vi "ChoixFiltres.vi"(1 "Ordre des filtres Avant":string[](array[string])=["Aucun filtre", "Filtre 1", "Filtre 2", "Filtre 3", "Filtre 4", ""]) -> (0 "Ordre des filtres Après":string[](array[string])=["Aucun filtre", "Filtre 1", "Filtre 2", "Filtre 3", "Filtre 4", ""])   [LabVIEW 2011]
panel:
  in  "Annuler":bool
  in  "OK":bool
  in  "Filtre 6":string
  in  "Filtre 5":string="Filtre 4"
  in  "Filtre 4":string="Filtre 3"
  in  "Filtre 3":string="Filtre 2"
  in  "Filtre 2":string="Filtre 1"
  in  "Filtre 1":string="Aucun filtre"
  # "Appuyer sur \"ENTER\" pour confirmer\nla modification de l'étiquette de filtre."
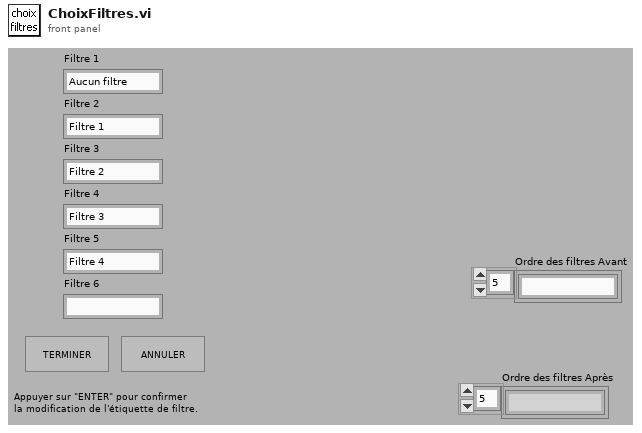
[diagram p1: front panel]
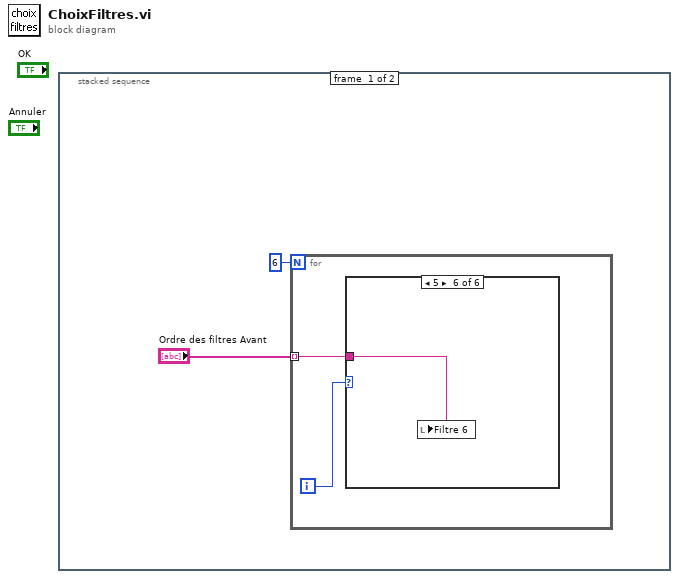
[diagram p0: block diagram]
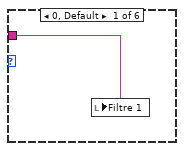
[diagram p2: hidden frame]
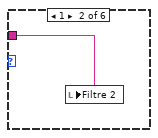
[diagram p3: hidden frame]
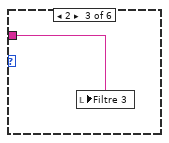
[diagram p4: hidden frame]
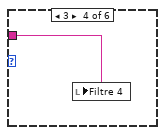
[diagram p5: hidden frame]
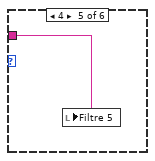
[diagram p6: hidden frame]
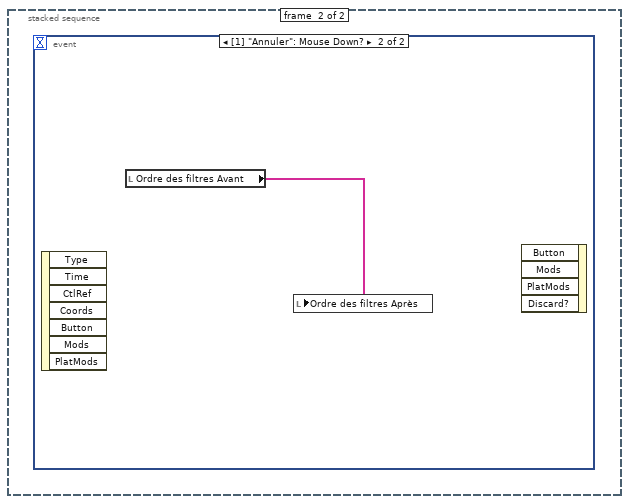
[diagram p7: hidden frame]
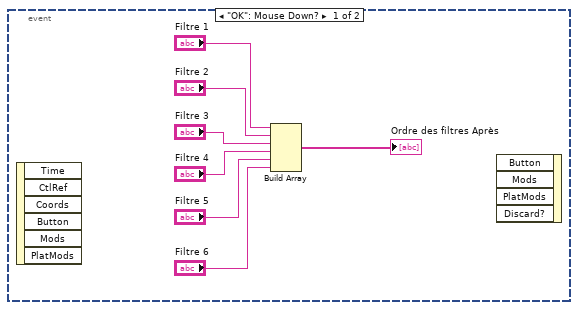
[diagram p8: hidden frame]
diagram:
  n1 = stacked-sequence {
    frame #0 {
      n2 = for {
        N: 6 -> [_]
        tunnel: "Ordre des filtres Avant" -> [w3] mode=indexing
        i -> [w4]
        n3 = case shown="5" w4 {
          tunnel: w3 -> [w5 w6 w7 w8 w9 w10]
          frame 0, Default {
            n4 = local write "Filtre 1"(w5) -> ()
          }
          frame 1 {
            n5 = local write "Filtre 2"(w6) -> ()
          }
          frame 2 {
            n6 = local write "Filtre 3"(w7) -> ()
          }
          frame 3 {
            n7 = local write "Filtre 4"(w8) -> ()
          }
          frame 4 {
            n8 = local write "Filtre 5"(w9) -> ()
          }
          frame 5 {
            n9 = local write "Filtre 6"(w10) -> ()
          }
        }
      }
    }
    frame #1 {
      n10 = event shown="[1] \"Annuler\": Mouse Down?" {
        selector: _ -> [_ _]
        dyn-events: _ -> [_ _]
        timeout: _ -> [_ _]
        event "OK": Mouse Down? {
          n11 = event-data() -> ()  [unwired: 1 in, 6 out]
          n12 = Build Array("Filtre 1", "Filtre 2", "Filtre 3", "Filtre 4", "Filtre 5", "Filtre 6") -> (→"Ordre des filtres Après":string[])
          n13 = event-data() -> ()  [unwired: 5 in, 1 out]
        }
        event "Annuler": Mouse Down? {
          n14 = event-data() -> ()  [unwired: 1 in, 7 out]
          n15 = local read "Ordre des filtres Avant"() -> (w18:string[])
          n16 = local write "Ordre des filtres Après"(w18) -> ()
          n17 = event-data() -> ()  [unwired: 5 in, 1 out]
        }
      }
    }
  }
